vi "DC izvor.vi"() -> ()   [LabVIEW 2019]
uses:
  4x7 segment controls/top-segment.ctl
  4x7 segment controls/left-segment.ctl
  4x7 segment controls/rigt-segment.ctl
  4x7 segment controls/mid-segment.ctl
  4x7 segment controls/bottom-segment.ctl
  4x7 segment controls/decimal.ctl
  Analog multimeter/Controls/Enum_states.ctl
  <vilib>/numeric/Random Number (Range) DBL.vi
  Globals/Global message.vi
  Globals/CH1.vi
  Globals/CH2.vi
  Globals/CH3.vi
  Globals/CH4.vi
  Globals/CH5.vi
panel:
  in  "Gaussian noise":bool
  in  "Output channel current":T1(ring)
  in  "Output channel voltage":T1(ring)
  out "CV":bool
  out "CC":bool
  out "Power":bool
  in  "Stop Button":bool
  in  "Current coarse":dbl(knob) scale=0.0..5.0
  in  "Current fine":dbl(knob) scale=-0.5..0.5
  in  "Voltage fine":dbl(knob) scale=-1.0..1.0
  in  "Voltage coarse":dbl(knob) scale=0.0..30.0
  out "?":T8
  out "?":T8
  # "Voltage channel"
  # "Current channel"
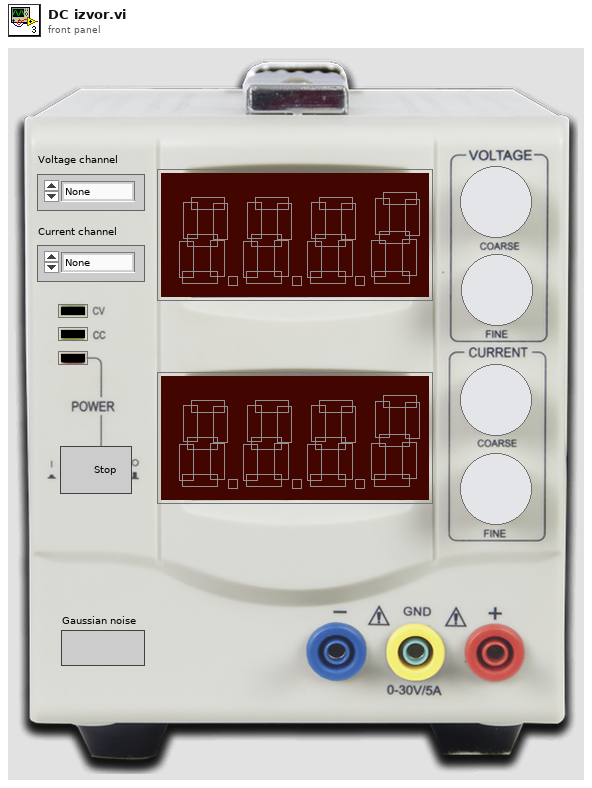
[diagram p1: front panel]
types:
  T1 = enum16{"None", "CH 1", "CH 2", "CH 3", "CH 4", "CH 5"}
  T2 = typedef "top-segment.ctl" = bool
  T3 = typedef "left-segment.ctl" = bool
  T4 = typedef "rigt-segment.ctl" = bool
  T5 = typedef "mid-segment.ctl" = bool
  T6 = typedef "bottom-segment.ctl" = bool
  T7 = typedef "decimal.ctl" = bool
  T8 = cluster{"1":cluster{"1":T2, "2":T3, "3":T4, "4":T5, "5":T3, "6":T4, "7":T6}, "2":cluster{"1":T2, "2":T3, "3":T4, "4":T5, "5":T3, "6":T4, "7":T6}, "3":cluster{"1":T2, "2":T3, "3":T4, "4":T5, "5":T3, "6":T4, "7":T6}, "4":cluster{"1":T2, "2":T3, "3":T4, "4":T5, "5":T3, "6":T4, "7":T6}, T7, T7, T7}
  T9 = cluster{"Voltage":dbl, "Current":dbl, "Message":string}
  T10 = typedef "Enum_states.ctl" = enum16{"Initialize", "Run", "Load", "Stop"}
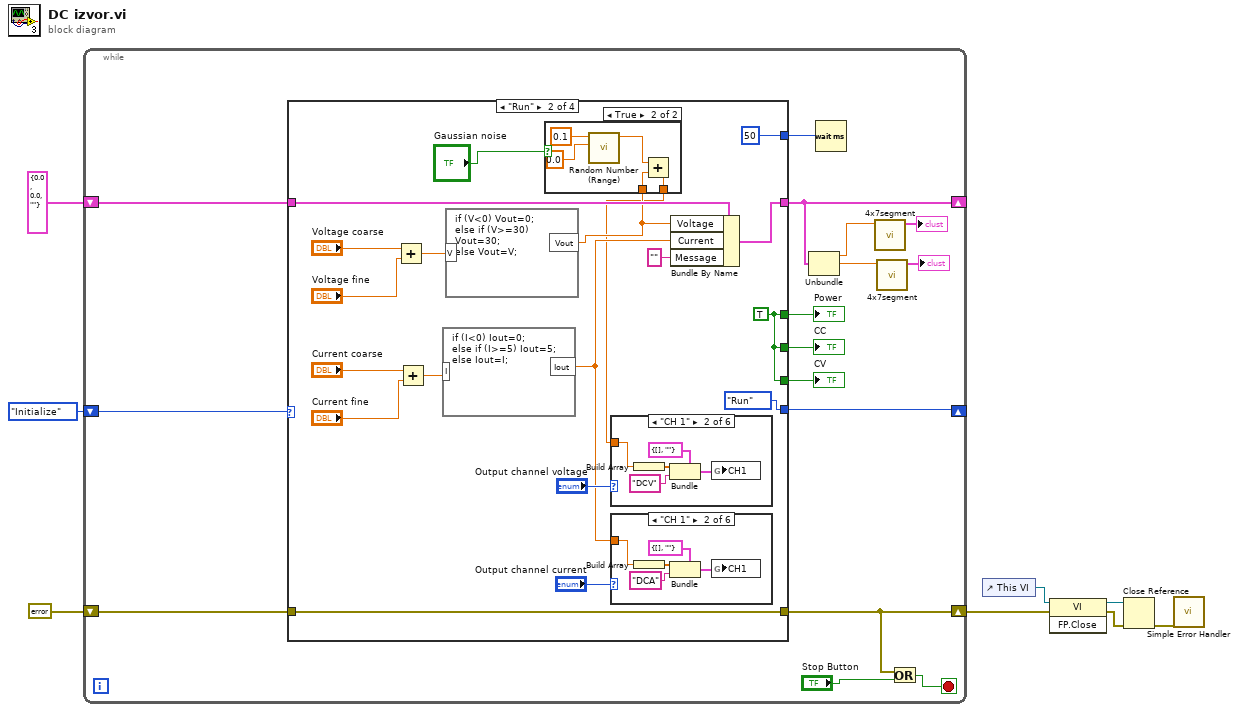
[diagram p0: block diagram]
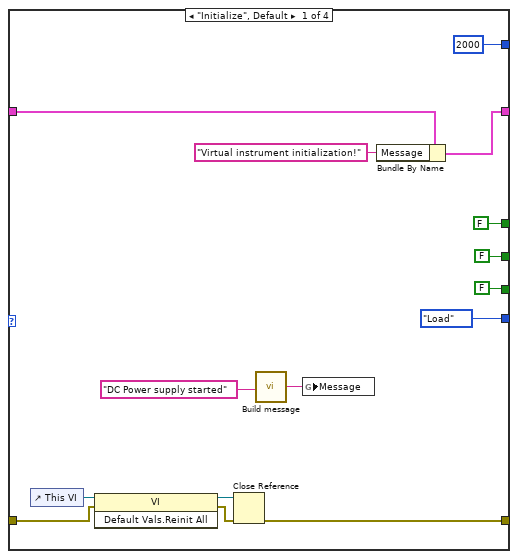
[diagram p2: hidden frame]
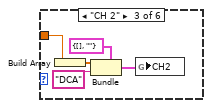
[diagram p5: hidden frame]
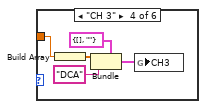
[diagram p6: hidden frame]
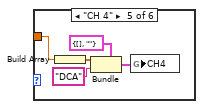
[diagram p7: hidden frame]
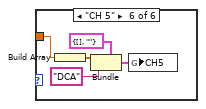
[diagram p8: hidden frame]
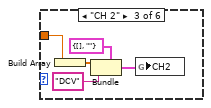
[diagram p10: hidden frame]
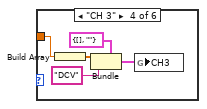
[diagram p11: hidden frame]
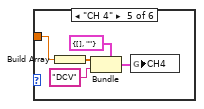
[diagram p12: hidden frame]
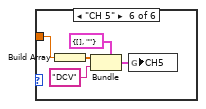
[diagram p13: hidden frame]
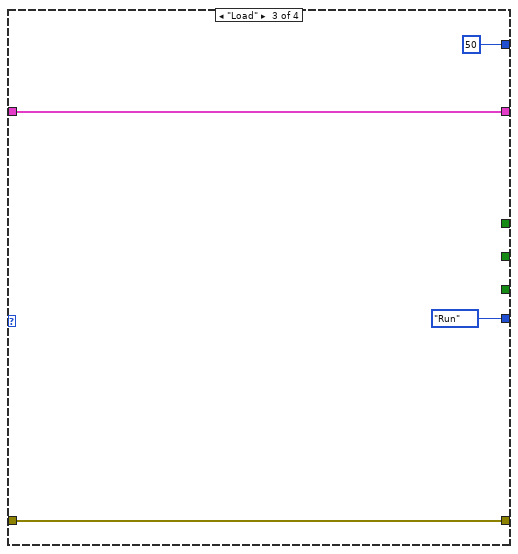
[diagram p14: hidden frame]
diagram:
  n1 = while {
    shift-right: [w22] -> w6
    shift-left: errorcluster {"status"=FALSE, "code"=0, "source"=""} ("error constant") -> [w24]
    shift-right: [w18] -> _
    shift-left: T9 {"Voltage"=0.0, "Current"=0.0, "Message"=""} -> [w21]
    shift-right: [w19] -> _
    shift-left: Enum_states."Initialize" ("Enum") -> [w20]
    stop <- w23 stop-if-true
    n2 = case shown="\"Run\"" w20 {
      selector: w20 -> [_ _ _ w119]
      tunnel: w24 -> [w36 w58 w117 w121]
      tunnel: [w30 w58 w117 w121] -> w22
      tunnel: w21 -> [w32 w54 w115 w120]
      tunnel: [w31 w56 w115 w120] -> w18
      tunnel: [Enum_states."Load" ("Enum") Enum_states."Run" ("Enum") Enum_states."Run" ("Enum") w119] -> w19
      tunnel: [u32 2000 ("milliseconds to wait") u32 50 ("milliseconds to wait") u32 50 ("milliseconds to wait") _] -> w17
      tunnel: [FALSE w43 _ _] -> w11
      tunnel: [FALSE w43 _ _] -> w10
      tunnel: [FALSE w43 _ _] -> w9
      frame "Initialize", Default {
        n3 = control-ref of="This VI"() -> (w39:refnum<vi>)
        n4 = invoke class="VI" method="Default Vals.Reinit All"(reference=w39, error in=w36) -> (reference out=w38:refnum<vi>, error out=w37:errorcluster)  [unwired: 1 in, 1 out]
        n5 = Close Reference(reference=w38, error in (no error)=w37) -> (error out=w30:errorcluster)
        n6 = call "Build message.vi"("Input string"="DC Power supply started") -> ("Output string"=w25:string)
        n7 = global write "Global message.vi" "Message"(w25) -> ()
        n8 = Bundle By Name(cluster=w32, "Message"="Virtual instrument initialization!") -> (w31:T9)
      }
      frame "Run" {
        w43 = TRUE
        n9 = Add(x="Voltage coarse", y="Voltage fine") -> (x+y=w49:dbl)
        n10 = Add(x="Current coarse", y="Current fine") -> (x+y=w47:dbl)
        n11 = formula code="if (I<0) Iout=0;\nelse if (I>=5) Iout=5;\nelse Iout=I;"("I"=w47) -> ("Iout"=w44:dbl)
        n12 = formula code="if (V<0) Vout=0;\nelse if (V>=30) Vout=30;\nelse Vout=V;"("V"=w49) -> ("Vout"=w41:dbl)
        n13 = case shown="True" "Gaussian noise" {
          tunnel: w41 -> [w59 w61]
          tunnel: [w59 w60] -> w40
          frame False {
          }
          frame True {
            n14 = call-poly <vilib>:"Random Number (Range).vi"("lower bound (0)"=0.0, "upper bound (100)"=0.1) -> ("number"=w62:dbl)  [unwired: 9 in]
            n15 = Add(x=w62, y=w61) -> (x+y=w60:dbl)
          }
        }
        n16 = case shown="\"CH 1\"" "Output channel voltage" {
          tunnel: w40 -> [_ w93 w97 w102 w107 w112]
          frame "None", Default {
          }
          frame "CH 1" {
            n17 = Build Array(w93) -> (w92:dbl[])
            n18 = Bundle(cluster=cluster{"CH1 Array":dbl[], "CH1 Message":string} {"CH1 Array"=[], "CH1 Message"=""} ("CH1"), "CH1 Array"=w92, "CH1 Message"="DCV") -> (w91:cluster{"CH1 Array":dbl[], "CH1 Message":string})
            n19 = global write "CH1.vi" "CH1"(w91) -> ()
          }
          frame "CH 2" {
            n20 = Build Array(w97) -> (w98:dbl[])
            n21 = Bundle(cluster=cluster{"CH1 Array":dbl[], "CH1 Message":string} {"CH1 Array"=[], "CH1 Message"=""} ("CH1"), "CH1 Array"=w98, "CH1 Message"="DCV") -> (w96:cluster{"CH1 Array":dbl[], "CH1 Message":string})
            n22 = global write "CH2.vi" "CH2"(w96) -> ()
          }
          frame "CH 3" {
            n23 = Build Array(w102) -> (w103:dbl[])
            n24 = Bundle(cluster=cluster{"CH1 Array":dbl[], "CH1 Message":string} {"CH1 Array"=[], "CH1 Message"=""} ("CH1"), "CH1 Array"=w103, "CH1 Message"="DCV") -> (w101:cluster{"CH1 Array":dbl[], "CH1 Message":string})
            n25 = global write "CH3.vi" "CH3"(w101) -> ()
          }
          frame "CH 4" {
            n26 = Build Array(w107) -> (w108:dbl[])
            n27 = Bundle(cluster=cluster{"CH1 Array":dbl[], "CH1 Message":string} {"CH1 Array"=[], "CH1 Message"=""} ("CH1"), "CH1 Array"=w108, "CH1 Message"="DCV") -> (w106:cluster{"CH1 Array":dbl[], "CH1 Message":string})
            n28 = global write "CH4.vi" "CH4"(w106) -> ()
          }
          frame "CH 5" {
            n29 = Build Array(w112) -> (w113:dbl[])
            n30 = Bundle(cluster=cluster{"CH1 Array":dbl[], "CH1 Message":string} {"CH1 Array"=[], "CH1 Message"=""} ("CH1"), "CH1 Array"=w113, "CH1 Message"="DCV") -> (w111:cluster{"CH1 Array":dbl[], "CH1 Message":string})
            n31 = global write "CH5.vi" "CH5"(w111) -> ()
          }
        }
        n32 = case shown="\"CH 1\"" "Output channel current" {
          tunnel: w44 -> [_ w68 w72 w77 w82 w87]
          frame "None", Default {
          }
          frame "CH 1" {
            n33 = Build Array(w68) -> (w67:dbl[])
            n34 = Bundle(cluster=cluster{"CH1 Array":dbl[], "CH1 Message":string} {"CH1 Array"=[], "CH1 Message"=""} ("CH1"), "CH1 Array"=w67, "CH1 Message"="DCA") -> (w66:cluster{"CH1 Array":dbl[], "CH1 Message":string})
            n35 = global write "CH1.vi" "CH1"(w66) -> ()
          }
          frame "CH 2" {
            n36 = Build Array(w72) -> (w73:dbl[])
            n37 = Bundle(cluster=cluster{"CH1 Array":dbl[], "CH1 Message":string} {"CH1 Array"=[], "CH1 Message"=""} ("CH1"), "CH1 Array"=w73, "CH1 Message"="DCA") -> (w71:cluster{"CH1 Array":dbl[], "CH1 Message":string})
            n38 = global write "CH2.vi" "CH2"(w71) -> ()
          }
          frame "CH 3" {
            n39 = Build Array(w77) -> (w78:dbl[])
            n40 = Bundle(cluster=cluster{"CH1 Array":dbl[], "CH1 Message":string} {"CH1 Array"=[], "CH1 Message"=""} ("CH1"), "CH1 Array"=w78, "CH1 Message"="DCA") -> (w76:cluster{"CH1 Array":dbl[], "CH1 Message":string})
            n41 = global write "CH3.vi" "CH3"(w76) -> ()
          }
          frame "CH 4" {
            n42 = Build Array(w82) -> (w83:dbl[])
            n43 = Bundle(cluster=cluster{"CH1 Array":dbl[], "CH1 Message":string} {"CH1 Array"=[], "CH1 Message"=""} ("CH1"), "CH1 Array"=w83, "CH1 Message"="DCA") -> (w81:cluster{"CH1 Array":dbl[], "CH1 Message":string})
            n44 = global write "CH4.vi" "CH4"(w81) -> ()
          }
          frame "CH 5" {
            n45 = Build Array(w87) -> (w88:dbl[])
            n46 = Bundle(cluster=cluster{"CH1 Array":dbl[], "CH1 Message":string} {"CH1 Array"=[], "CH1 Message"=""} ("CH1"), "CH1 Array"=w88, "CH1 Message"="DCA") -> (w86:cluster{"CH1 Array":dbl[], "CH1 Message":string})
            n47 = global write "CH5.vi" "CH5"(w86) -> ()
          }
        }
        n48 = Bundle By Name(cluster=w54, "Voltage"=w41, "Current"=w44, "Message"="") -> (w56:T9)
      }
      frame "Load" {
      }
      frame "Stop" {
      }
    }
    "Power" <- w9
    "CC" <- w11
    "CV" <- w10
    n49 = Unbundle(w18) -> ("Voltage"=w15:dbl, "Current"=w14:dbl)  [unwired: 1 out]
    n50 = Wait (ms)(milliseconds to wait=w17) -> ()  [unwired: 1 out]
    n51 = call "4x7segment.vi"("Numeric Control"=w15) -> (3:→"?":T8)  [unwired: 10 in]
    n52 = call "4x7segment.vi"("Numeric Control"=w14) -> (3:→"?":T8)  [unwired: 10 in]
    n53 = Or(x=w22, y="Stop Button") -> (x .or. y?=w23:bool)
  }
  n54 = control-ref of="This VI"() -> (w3:refnum<vi>)
  n55 = invoke class="VI" method="FP.Close"(reference=w3, error in=w6) -> (reference out=w1:refnum<vi>, error out=w2:errorcluster)  [unwired: 1 in, 1 out]
  n56 = Close Reference(reference=w1, error in (no error)=w2) -> (error out=w5:errorcluster)
  n57 = call <vilib>:"Simple Error Handler.vi"("error in (no error)"=w5) -> ()  [unwired: 4 in, 5 out]
